vi "Main Code.vi"() -> ()   [LabVIEW 2017]
uses:
  <vilib>/MakerHub/LINX/Public/Peripherals/Analog/Analog Read 1 Chan.vi
  <vilib>/MakerHub/LINX/Public/Peripherals/Digital/Digital Write N Chans.vi
  <vilib>/MakerHub/LINX/Public/Peripherals/Analog/Analog Read N Chans.vi
  <vilib>/MakerHub/LINX/Private/Local IO/LinxDigitalWrite.vi
  <vilib>/MakerHub/LINX/Public/Utilities/Check Channel.vi
  <vilib>/MakerHub/LINX/Private/Local IO/LinxAnalogRead.vi
  <vilib>/MakerHub/LINX/Public/Utilities/Open Serial.vi
  <vilib>/MakerHub/LINX/Private/Utilties/Generate Error.vi
  <vilib>/MakerHub/LINX/LMH-LINX.lvlib
panel:
  out "Power":dbl
  out "current":dbl
  out "max val 2":dbl
  out "Voltage 2":dbl
  out "loop":i32
  in  "max val":dbl
  out "Voltage":dbl
  in  "Stop Button":bool
  out "Loop Rate (Hz)":u32
  in  "relay":dbl
  out "element":dbl
  out "Input voltage":dbl
  in  "Serial Port":refnum<visa-resource-name>
  # "EE-314L Projet"
  # "Auto tap transformer"
  # "Check"
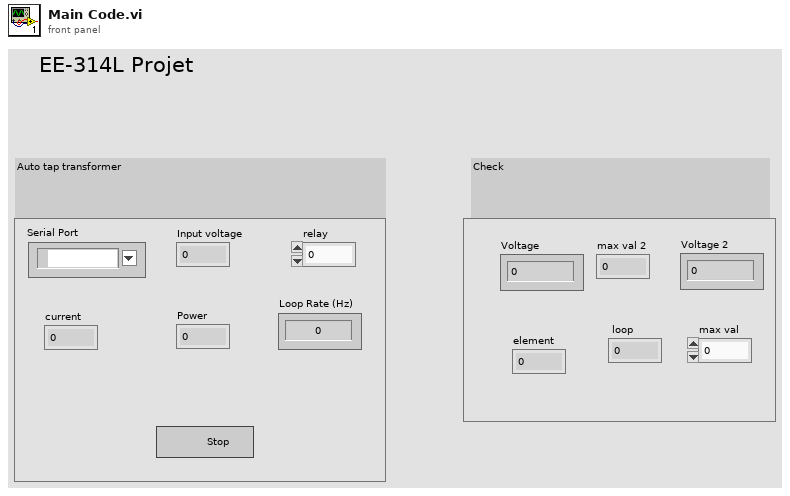
[diagram p1: front panel]
types:
  T1 = typedef "LMH-LINX.lvlib/LINX Ref.ctl" = cluster{"IO":T2, "Interface":T3, "LINX Device Config":T4}
  T2 = typedef "LMH-LINX.lvlib/Platform.ctl" = enum16{"Remote", "Local"}
  T3 = typedef "LMH-LINX.lvlib/Interface.ctl" = enum16{"Serial", "TCP"}
  T4 = typedef "LMH-LINX.lvlib/Device.lvlib/LINX Device Config.ctl" = cluster{"Interface":T3, "COM Port":refnum<visa-resource-name>, "TCP Configuration":T5, "Device Family":u8, "Device ID":u8, "Device Name":string, "TCP Ref":refnum<k5>, "Channels":T6}
  T5 = typedef "LMH-LINX.lvlib/Device.lvlib/TCP Config.ctl" = cluster{"IP Address":string, "Port":u16}
  T6 = typedef "LMH-LINX.lvlib/Channels.ctl" = cluster{"DI":u8[], "DO":u8[], "AI":u8[], "AO":u8[], "PWM":u8[], "QE":u8[], "UART":u8[], "I2C 2":u8[], "SPI":u8[], "CAN":u8[], "Servo":u8[], "AI Ref (V)":dbl, "AI Resolution (Bits)":u8, "AO Ref (V)":dbl, "AO Resolution (Bits)":u8}
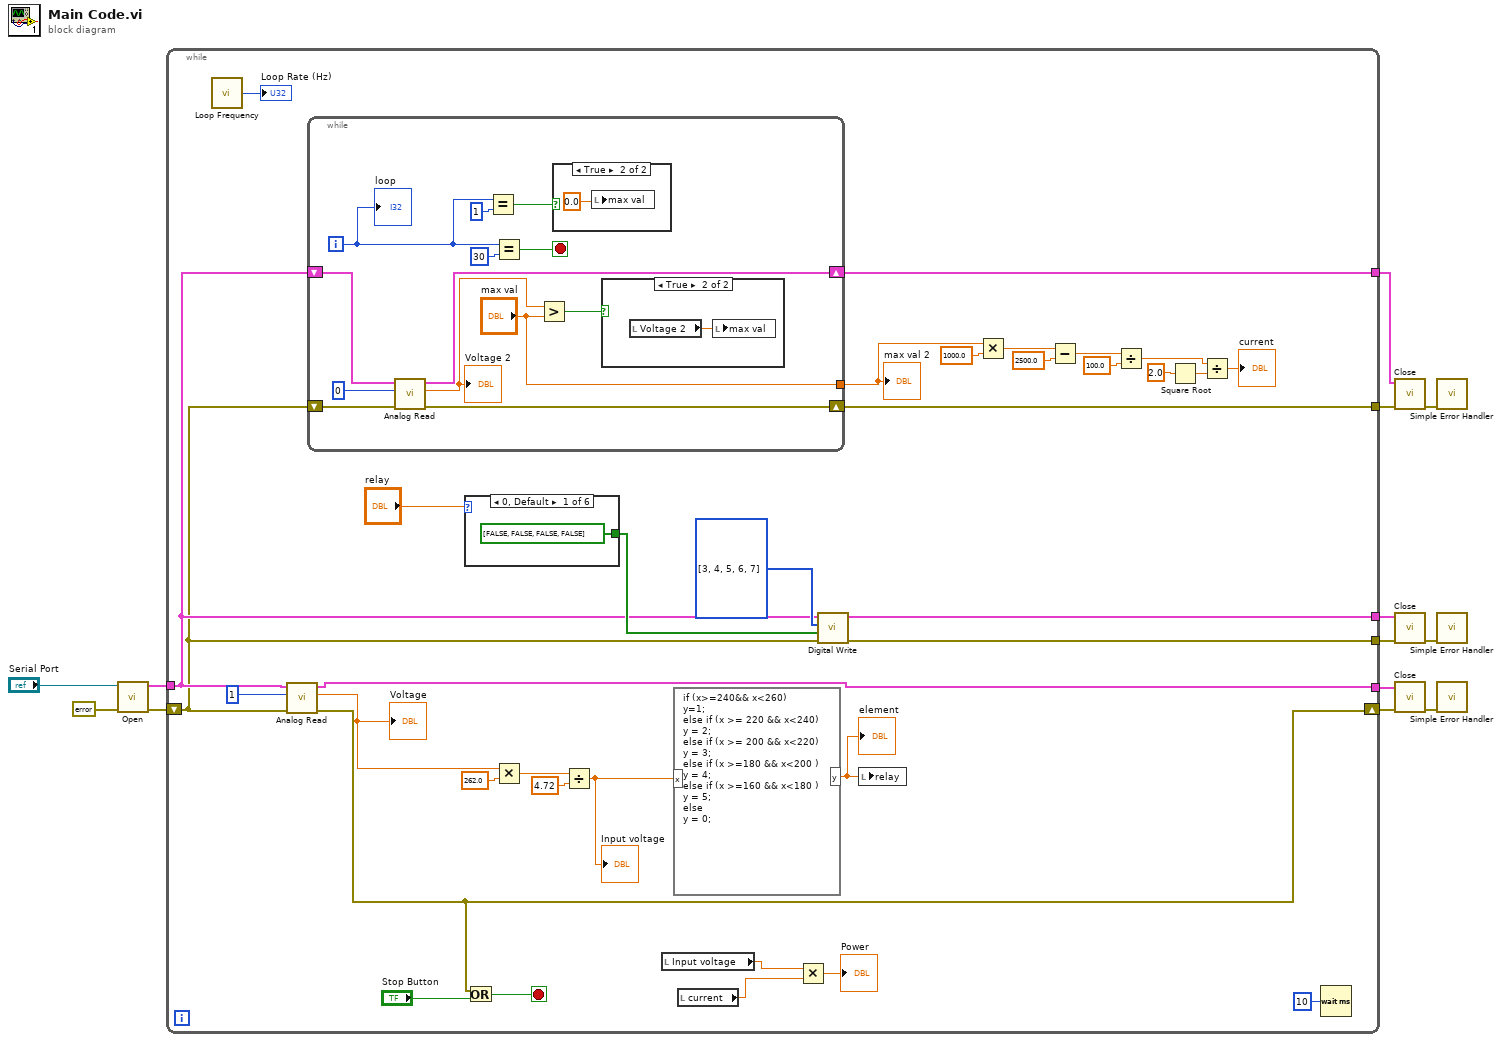
[diagram p0: block diagram]
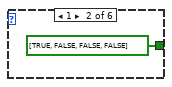
[diagram p4: hidden frame]
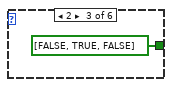
[diagram p5: hidden frame]
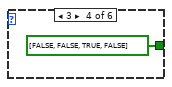
[diagram p6: hidden frame]
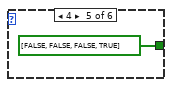
[diagram p7: hidden frame]
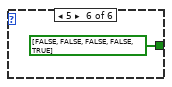
[diagram p8: hidden frame]
diagram:
  n1 = call-poly <vilib>:"Open.vi"("Error In"=errorcluster {"status"=FALSE, "code"=0, "source"=""}, "Serial Port"="Serial Port") -> ("Error Out"=w12:errorcluster, "LINX Resource"=w13:T1)  [unwired: 7 in, 1 out]
  n2 = while {
    tunnel: w13 -> [w31]
    tunnel: [w45] -> w11
    shift-right: [w44] -> w10
    shift-left: w12 -> [w30]
    tunnel: [w42] -> w6
    tunnel: [w41] -> w5
    tunnel: [w29] -> w2
    tunnel: [w28] -> w1
    stop <- w48 stop-if-true
    n3 = call <vilib>:"Loop Frequency.vi"() -> ("Loop Rate (Hz)"=→"Loop Rate (Hz)":u32)
    n4 = call-poly <vilib>:"Analog Read.vi"("Error In"=w30, "Analog Channel"=u8 1, "LINX Resource"=w31) -> ("Error Out"=w44:errorcluster, "Voltage"=w32:dbl, "LINX Resource"=w45:T1)  [unwired: 5 in, 1 out]
    "Voltage" <- w32
    n5 = while {
      shift-right: [w59] -> w28
      shift-left: w30 -> [w61]
      shift-right: [w58] -> w29
      shift-left: w31 -> [w60]
      tunnel: ["max val"] -> w18
      i -> [w52]
      stop <- w55 stop-if-true
      n6 = call-poly <vilib>:"Analog Read.vi"("Error In"=w61, "Analog Channel"=u8 0, "LINX Resource"=w60) -> ("Error Out"=w59:errorcluster, "Voltage"=w53:dbl, "LINX Resource"=w58:T1)  [unwired: 5 in, 1 out]
      "Voltage 2" <- w53
      n7 = Equal?(x=w52, y=1) -> (x = y?=w50:bool)
      n8 = Equal?(x=w52, y=30) -> (x = y?=w55:bool)
      n9 = Greater?(x=w53, y="max val") -> (0:w54:bool)
      n10 = case shown="True" w50 {
        frame False {
        }
        frame True {
          n11 = local write "max val"(0.0 ("max val")) -> ()
        }
      }
      n12 = case shown="True" w54 {
        frame False {
        }
        frame True {
          n13 = local read "Voltage 2"() -> (w63:dbl)
          n14 = local write "max val"(w63) -> ()
        }
      }
      "loop" <- w52
    }
    "max val 2" <- w18
    n15 = case shown="0, Default" "relay" {
      tunnel: [bool[] [FALSE, FALSE, FALSE, FALSE] ("Values") bool[] [TRUE, FALSE, FALSE, FALSE] ("Values") bool[] [FALSE, TRUE, FALSE] ("Values") bool[] [FALSE, FALSE, TRUE, FALSE] ("Values") bool[] [FALSE, FALSE, FALSE, TRUE] ("Values") bool[] [FALSE, FALSE, FALSE, FALSE, TRUE] ("Values")] -> w40
      frame 0, Default {
      }
      frame 1 {
      }
      frame 2 {
      }
      frame 3 {
      }
      frame 4 {
      }
      frame 5 {
      }
    }
    n16 = Or(x=w44, y="Stop Button") -> (x .or. y?=w48:bool)
    n17 = Multiply(x=w32, y=262.0) -> (x*y=w37:dbl)
    n18 = Divide(x=w37, y=4.72) -> (x/y=w35:dbl)
    "Input voltage" <- w35
    n19 = local read "Input voltage"() -> (w16:dbl)
    n20 = formula code="if (x>=240&& x<260)\ny=1;\nelse if (x >= 220 && x<240)\ny = 2;\nelse if (x >= 200 && x<220)\ny = 3;\nelse if (x >=180 && x<200 )\ny = 4;\nelse if (x >=160 && x<180 )\ny = 5;\nelse\ny = 0;"("x"=w35) -> ("y"=w34:dbl)
    "element" <- w34
    n21 = local read "current"() -> (w15:dbl)
    n22 = Multiply(x=w16, y=w15) -> (x*y=→"Power":dbl)
    n23 = call-poly <vilib>:"Digital Write.vi"("Error In"=w30, "Values"=w40, "DO Channels"=u8[] [3, 4, 5, 6, 7], "LINX Resource"=w31) -> ("Error Out"=w41:errorcluster, "LINX Resource"=w42:T1)  [unwired: 6 in]
    n24 = local write "relay"(w34) -> ()
    n25 = Multiply(x=w18, y=1000.0) -> (x*y=w23:dbl)
    n26 = Subtract(x=w23, y=2500.0) -> (x-y=w27:dbl)
    n27 = Divide(x=w27, y=100.0) -> (x/y=w24:dbl)
    n28 = Square Root(x=2.0) -> (sqrt(x)=w25:dbl)
    n29 = Divide(x=w24, y=w25) -> (x/y=→"current":dbl)
    n30 = Wait (ms)(milliseconds to wait=u32 10) -> ()  [unwired: 1 out]
  }
  n31 = call <vilib>:"Close.vi"("Error In"=w1, "LINX Resource"=w2) -> ("Error Out"=w3:errorcluster)  [unwired: 9 in]
  n32 = call <vilib>:"Close.vi"("Error In"=w5, "LINX Resource"=w6) -> ("Error Out"=w7:errorcluster)  [unwired: 9 in]
  n33 = call <vilib>:"Close.vi"("Error In"=w10, "LINX Resource"=w11) -> ("Error Out"=w8:errorcluster)  [unwired: 9 in]
  n34 = call <vilib>:"Simple Error Handler.vi"("error in (no error)"=w3) -> ()  [unwired: 4 in, 5 out]
  n35 = call <vilib>:"Simple Error Handler.vi"("error in (no error)"=w7) -> ()  [unwired: 4 in, 5 out]
  n36 = call <vilib>:"Simple Error Handler.vi"("error in (no error)"=w8) -> ()  [unwired: 4 in, 5 out]
